vi "Emitter.Test.vi"() -> ()   [LabVIEW 2016]
panel:
  in  "lockout_key":string
  in  "retcode":u16(ring) items=["0"=0, "1"=1, "100"=100, "101"=101, "102"=102, "200"=200, "201"=202, "300"=300, "301"=301, "302"=302, "303"=303, "304"=304, "305"=305, "306"=306, "307"=307, "308"=308, "309"=309, "400"=400, "500"=500, "501"=501, "502"=502, "999"=999]
  in  "msgop":i32(ring) items=["0"=0, "1"=1, "6"=6, "7"=7, "8"=8, "9"=9]
  in  "input json string":string="{\"values\":\"test\"}"
  in  "exchange name":u16(ring) items=["requests", "alerts"]
  in  "msgtype":i32(ring)=2 items=["2"=2, "3"=3, "4"=4]
  in  "routing key":string="broadcast"
  out "error out":errorcluster
  in  "error (in)":errorcluster
  in  "host name":string="higgsino.physics.ucsb.edu"
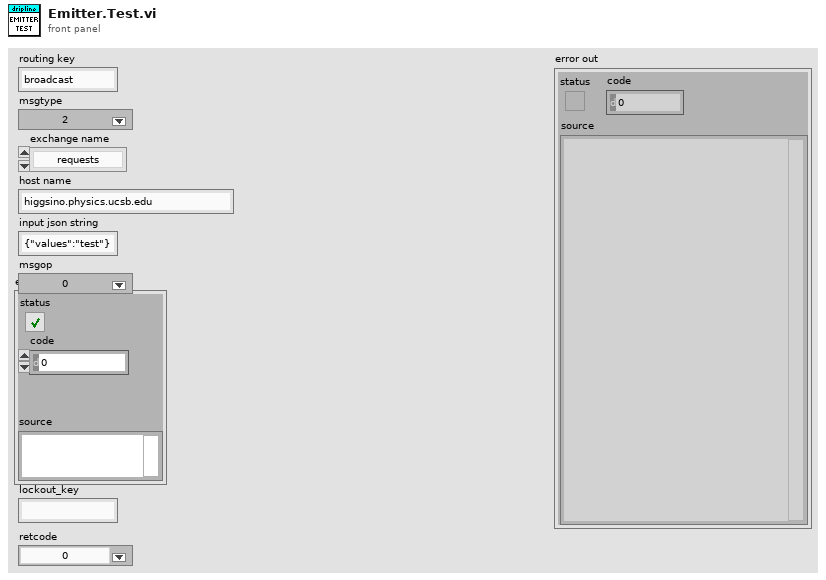
[diagram p1: front panel]
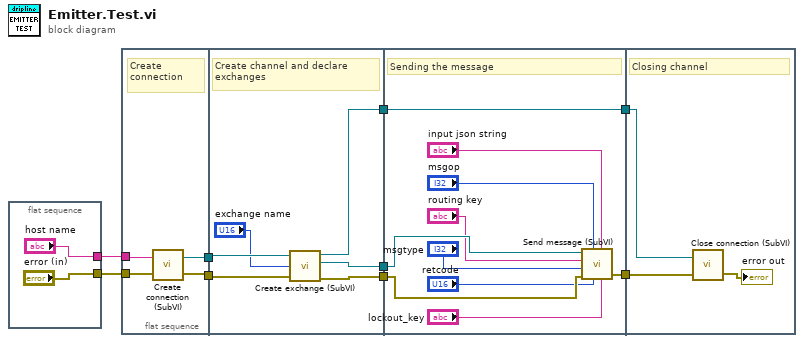
[diagram p0: block diagram]
diagram:
  n1 = flat-sequence {
    tunnel: ["error (in)"] -> w9
    tunnel: ["host name"] -> w8
    frame #0 {
    }
  }
  n2 = flat-sequence {
    tunnel: [w13] -> w7
    tunnel: [w14] -> w6
    tunnel: w8 -> [w15]
    tunnel: w9 -> [w12]
    tunnel: w7 -> [w21]
    tunnel: w6 -> [w20]
    tunnel: [w19] -> w5
    tunnel: [w18] -> w4
    tunnel: [w16] -> w1
    tunnel: w5 -> [w24]
    tunnel: w4 -> [w31]
    tunnel: [w28] -> w3
    tunnel: [w25] -> w2
    tunnel: w1 -> [w25]
    tunnel: w3 -> [w34]
    tunnel: w2 -> [w33]
    frame #0 {
      # "Create connection"
      n3 = call "Create connection (SubVI).vi"("error in (no error)"=w12, "host name"=w15) -> ("error out"=w14:errorcluster, "Connection out"=w13:refnum<class "Connection.lvclass">)
    }
    frame #1 {
      # "Create channel and declare exchanges"
      n4 = call "Create exchange (SubVI).vi"("Connection in"=w21, "exchange name"="exchange name", "error in (no error)"=w20) -> ("Connection out"=w16:refnum<class "Connection.lvclass">, "Exchange.lvclass"=w18:refnum<class "Exchange.lvclass">, "error out"=w19:errorcluster)  [unwired: 1 out]
    }
    frame #2 {
      # "Sending the message"
      n5 = call "Send message (SubVI).vi"("lockout_key"="lockout_key", "input json string"="input json string", "retcode"="retcode", "msgop"="msgop", "error in (no error)"=w24, "msgtype"="msgtype", "routing key"="routing key", "Exchange in"=w31) -> ("error out"=w28:errorcluster)  [unwired: 2 in, 1 out]
    }
    frame #3 {
      # "Closing channel"
      n6 = call "Close connection (SubVI).vi"("error in (no error)"=w34, "Connection in"=w33) -> ("error out"=→"error out":errorcluster)  [unwired: 1 in]
    }
  }
